vi "DUMMY SENDER 2.vi"() -> ()   [LabVIEW 2021]
panel:
  out "x+y":i32
  out "Waveform Graph 10":dynamicdata(graph)
  out "Numeric 3":dbl
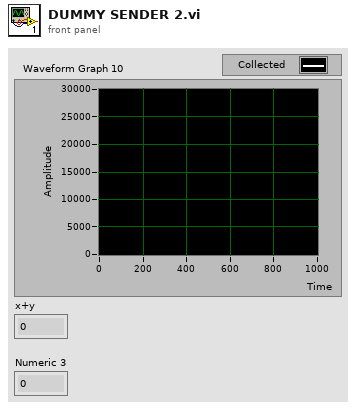
[diagram p1: front panel]
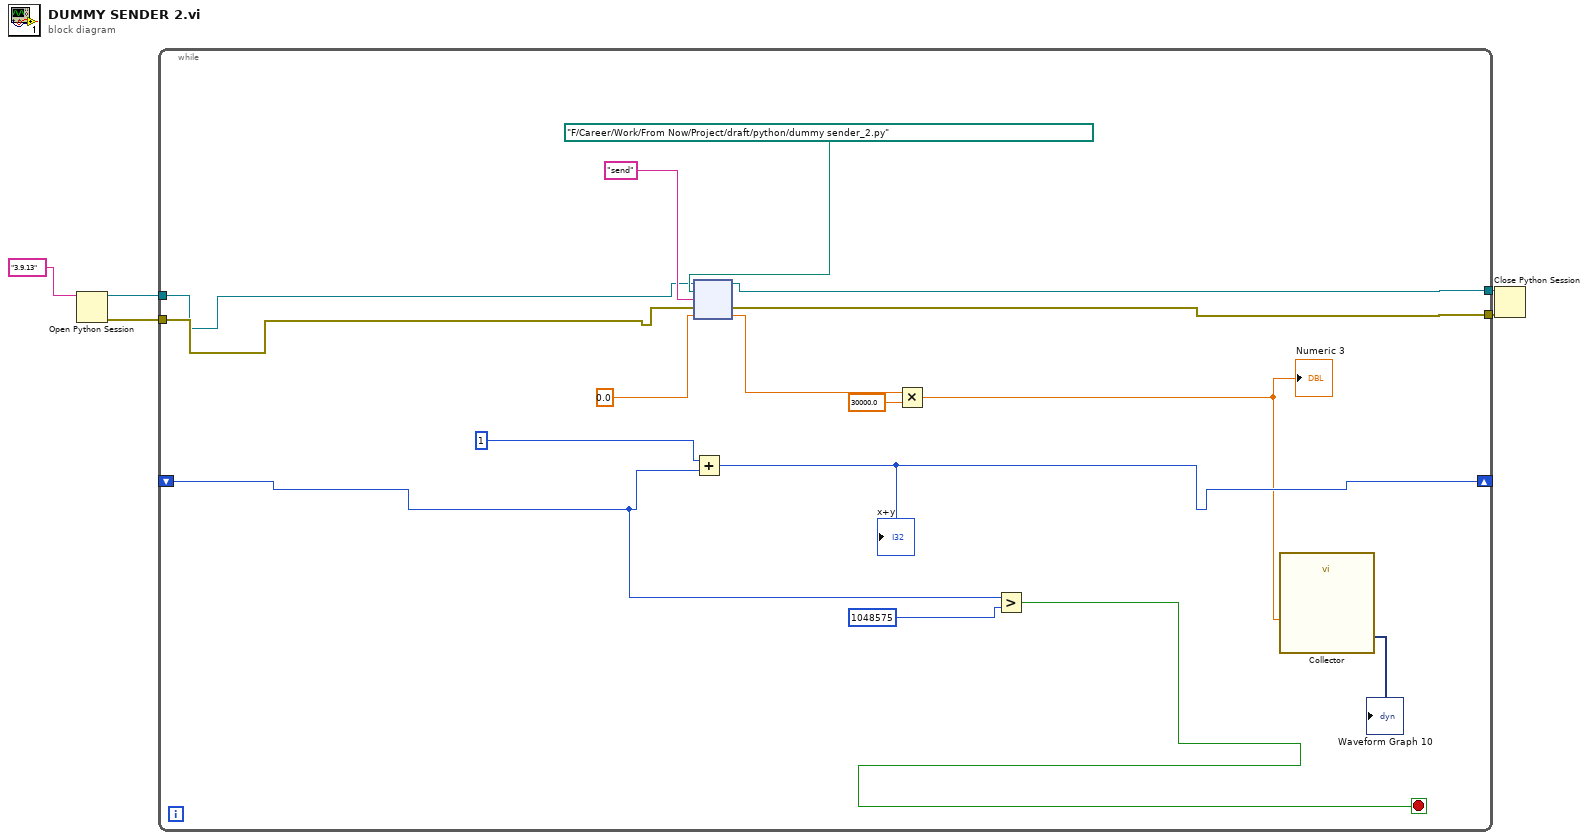
[diagram p0: block diagram]
diagram:
  n1 = Open Python Session(python version="3.9.13" ("Python version")) -> (session out=w4:refnum<k35>, error out=w3:errorcluster)  [unwired: 2 in]
  n2 = while {
    tunnel: w4 -> [w13]
    tunnel: w3 -> [w14]
    tunnel: [w16] -> w2
    tunnel: [w15] -> w1
    shift-right: [w10] -> _
    shift-left: _ -> [w11]
    stop <- w12 stop-if-true
    n3 = node(w13, path "F:/Career/Work/From Now/Project/draft/python/dummy sender_2.py" ("module path"), "send" ("function name"), w14, 0.0) -> (w16:refnum<k35>, w15:errorcluster, w8:dbl)  [unwired: 2 out]
    n4 = Add(x=1, y=w11) -> (x+y=w10:i32)
    "x+y" <- w10
    n5 = Multiply(x=w8, y=30000.0) -> (x*y=w6:dbl)
    "Numeric 3" <- w6
    n6 = Greater?(x=w11, y=1048575) -> (0:w12:bool)
    n7 = call "Collector"("Signals"=w6) -> ("Collected Signals"=→"Waveform Graph 10":dynamicdata)  [unwired: 9 in, 1 out]
  }
  n8 = Close Python Session(session in=w2, error in=w1) -> ()  [unwired: 1 out]
